vi "PUMP RAMP 2 (SubVI).vi"(0 "Dynamic Data":dynamicdata(waveform), 1 "Numeric":i16, 3 "Seq in":dbl[][](array[numeric])=[[20.0, 60.0, 40.0], [60.0, 40.0, 20.0], [100.0, 100.0, 100.0]], 4 "Device port":i32=7) -> (7 "Rate (g/s)":dbl, 10 "Weight (S1)":dbl, 11 "Step 2":i32, 12 "target reached":i32, 13 "x/y":dbl, 14 "Time (s)":dbl, 15 "bal_previous":i32, 17 "Target (g)":dbl, 18 "Waveform Chart 2":dynamicdata(graph))   [LabVIEW 2015]
uses:
  BERTTA.dll
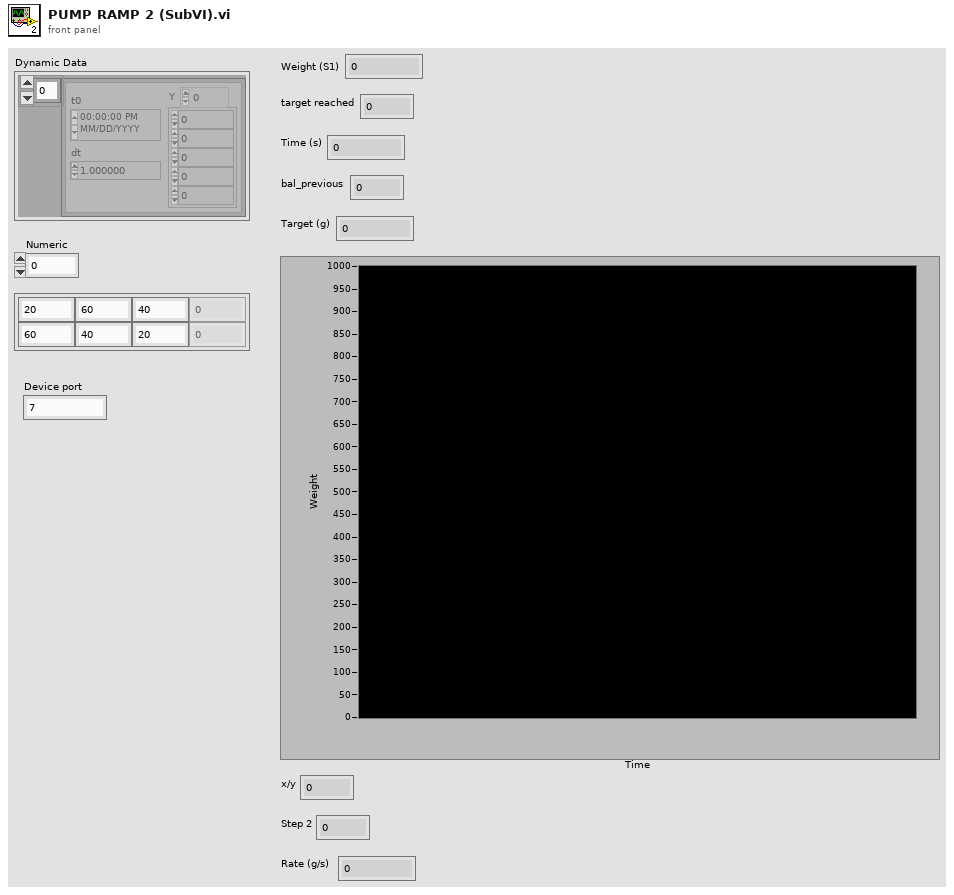
[diagram p1: front panel]
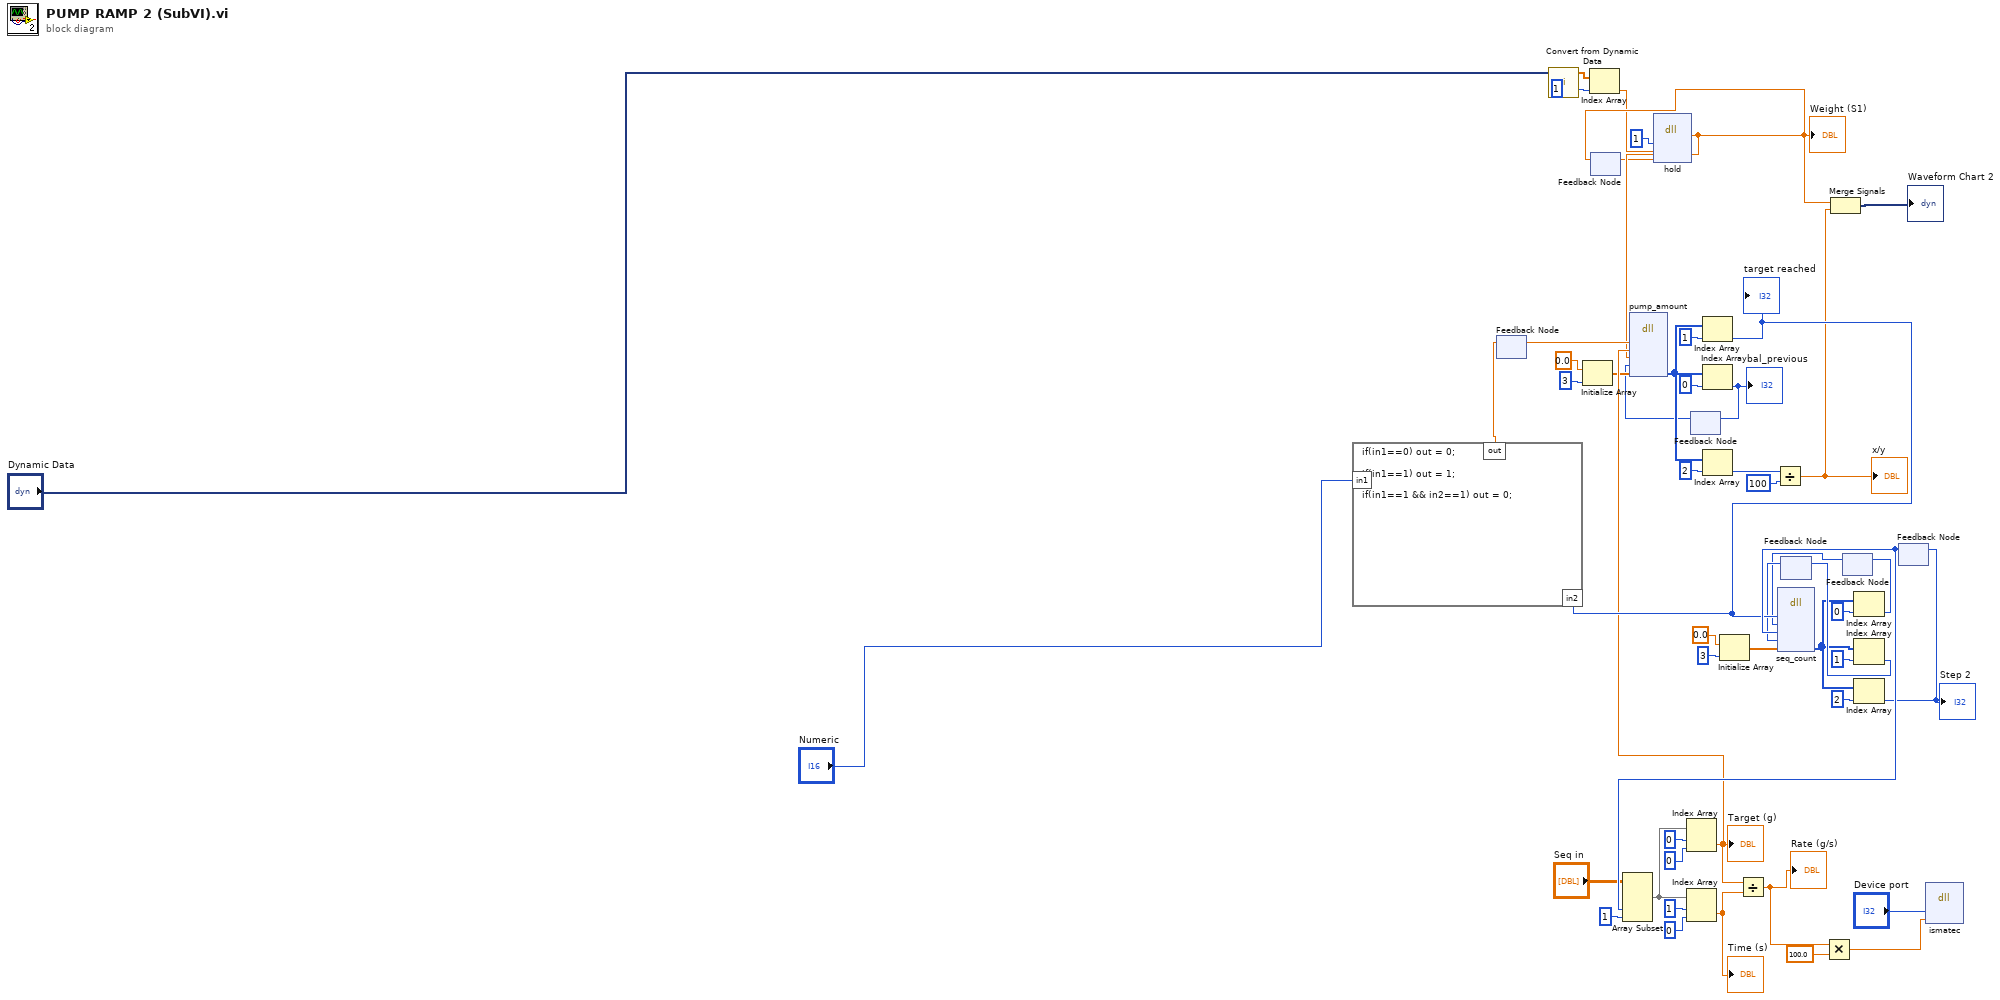
[diagram p0: block diagram]
diagram:
  n1 = feedback #1() -> (w47:dbl)  [unwired: 1 in]
  n2 = call "Convert from Dynamic Data"("Dynamic Data Type"="Dynamic Data") -> ("Array"=w14:dbl[])  [unwired: 3 in]
  n3 = Initialize Array(0.0 ("element"), 3 ("dimension size")) -> (w24:dbl[])
  n4 = Index Array(array=w14, index=1) -> (element=w15:dbl)
  n5 = feedback #2() -> (w16:dbl)  [unwired: 1 in]
  n6 = dll-call lib="C:/Users/xlaraser/Documents/Visual Studio 2017/Projects/Bertta/BERTTA/Debug/BERTTA.dll" fn="hold"("enable"=1, "in1"=w15, "in2"=w16) -> ("return type"=w27:dbl)  [unwired: 6 in, 2 out]
  "Weight (S1)" <- w27
  n7 = feedback-in #2(w27) -> ()
  n8 = feedback #3() -> (w21:i32)  [unwired: 1 in]
  n9 = Initialize Array(0.0 ("element"), 3 ("dimension size")) -> (w33:dbl[])
  n10 = feedback #4() -> (w41:i32)  [unwired: 1 in]
  n11 = feedback #5() -> (w40:i32)  [unwired: 1 in]
  n12 = feedback #6() -> (w49:i32)  [unwired: 1 in]
  n13 = Array Subset(array="Seq in", index (col)=w49, length (col)=1 ("length")) -> (w8:dbl[][])  [unwired: 2 in]
  n14 = Index Array(array=w8, index (row)=0, index (col)=0 ("disabled index (col)")) -> (element=w29:dbl)
  "Target (g)" <- w29
  n15 = dll-call lib="C:/Users/xlaraser/Documents/Visual Studio 2017/Projects/Bertta/BERTTA/Debug/BERTTA.dll" fn="pump_amount"("enable"=w47, "target"=w29, "bal"=w27, "bal_previous"=w21, "params"=w24) -> ("params"=w26:i32[])  [unwired: 8 in, 2 out]
  n16 = Index Array(array=w8, index (row)=1, index (col)=0 ("disabled index (col)")) -> (element=w12:dbl)
  "Time (s)" <- w12
  n17 = Index Array(array=w26, index=1) -> (element=w45:i32)
  "target reached" <- w45
  n18 = formula code="if(in1==0) out = 0;\n\nif(in1==1) out = 1;\n\nif(in1==1 && in2==1) out = 0;"("in1"="Numeric", "in2"=w45) -> ("out"=w46:dbl)
  n19 = feedback-in #1(w46) -> ()
  n20 = Index Array(array=w26, index=0) -> (element=w20:i32)
  "bal_previous" <- w20
  n21 = feedback-in #3(w20) -> ()
  n22 = Index Array(array=w26, index=2) -> (element=w30:i32)
  n23 = Divide(x=w29, y=w12) -> (x/y=w3:dbl)
  "Rate (g/s)" <- w3
  n24 = Divide(x=w30, y=100) -> (x/y=w31:dbl)
  "x/y" <- w31
  n25 = dll-call lib="C:/Users/xlaraser/Documents/Visual Studio 2017/Projects/Bertta/BERTTA/Debug/BERTTA.dll" fn="seq_count"("in1"=w45, "in2"=w40, "in3"=w49, "in4"=w41, "params"=w33) -> ("params"=w39:i32[])  [unwired: 8 in, 2 out]
  n26 = Multiply(x=w3, y=100.0) -> (x*y=w2:dbl)
  n27 = Merge Signals(w27, w31) -> (→"Waveform Chart 2":dynamicdata)
  n28 = Index Array(array=w39, index=0) -> (element=w42:i32)
  n29 = feedback-in #5(w42) -> ()
  n30 = Index Array(array=w39, index=1) -> (element=w43:i32)
  n31 = feedback-in #4(w43) -> ()
  n32 = Index Array(array=w39, index=2) -> (element=w48:i32)
  "Step 2" <- w48
  n33 = feedback-in #6(w48) -> ()
  n34 = dll-call lib="C:/Users/xlaraser/Documents/Visual Studio 2017/Projects/Bertta/BERTTA/Debug/BERTTA.dll" fn="ismatec"("port"="Device port", "speed"=w2) -> ()  [unwired: 6 in, 2 out]
